vi "correct depth etc 2016.vi"(2 "KPRO Culmulative \ntest report header 2":T1=["Measurement Time", "Current Absolute Depth (Uncorrected)", "Corrected Depth", "Depth Rate", "Flow", "Feet of Stainless Steel Used", "In line Pressure Sensor", "IK", "Corrected Headloss", "Atmospheric Pressure (global)", "Depth to Water Table (global)", "Height of Box (global)", "Resevoir Pressure (global)", "Seconds since Jan 1 1904", "Marker", "Downhole Pressure Sensor (ft/H20)", "Downhole Pressure Sensor (V)", "DHT Depth to Water", "DHT IK", "Current Relative Depth", "Previous Relative Depth"], 3 "New Stainless Feet":i32, 4 "Cumulative_data_in":dbl[][](array[numeric]) format="%.4f", 5 "First Absolute Depth":dbl format="%.2f", 6 "Incorrect Depth":dbl format="%.2f", 7 "Correct Depth":dbl format="%.2f") -> (1 "Cumulative_data_out":dbl[][](array[numeric]) format="%.4f")   [LabVIEW 2016]
uses:
  controls/KPro Header Control 1.ctl
  Kpro Globals.vi
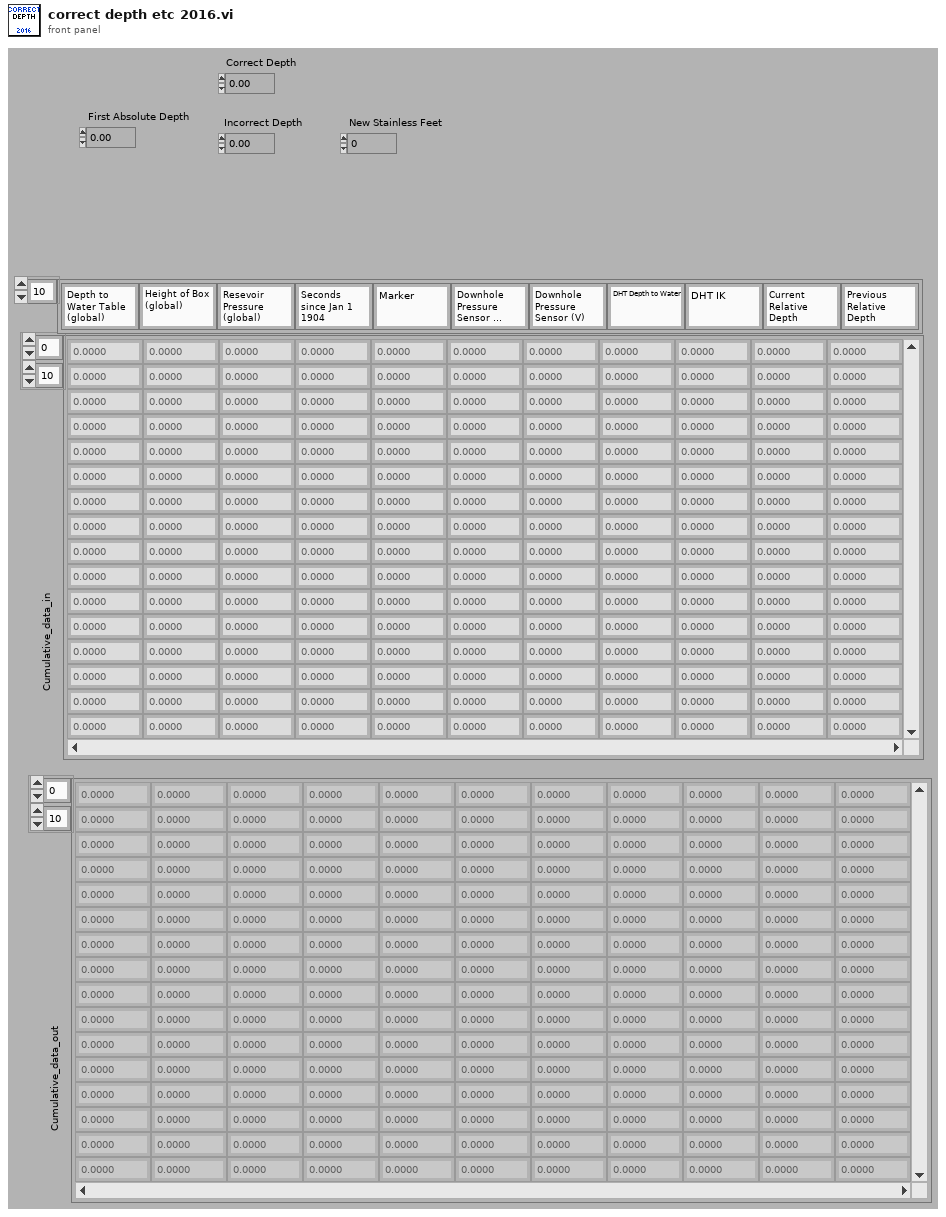
[diagram p1: front panel]
types:
  T1 = typedef "KPro Header Control 1.ctl" = string[]
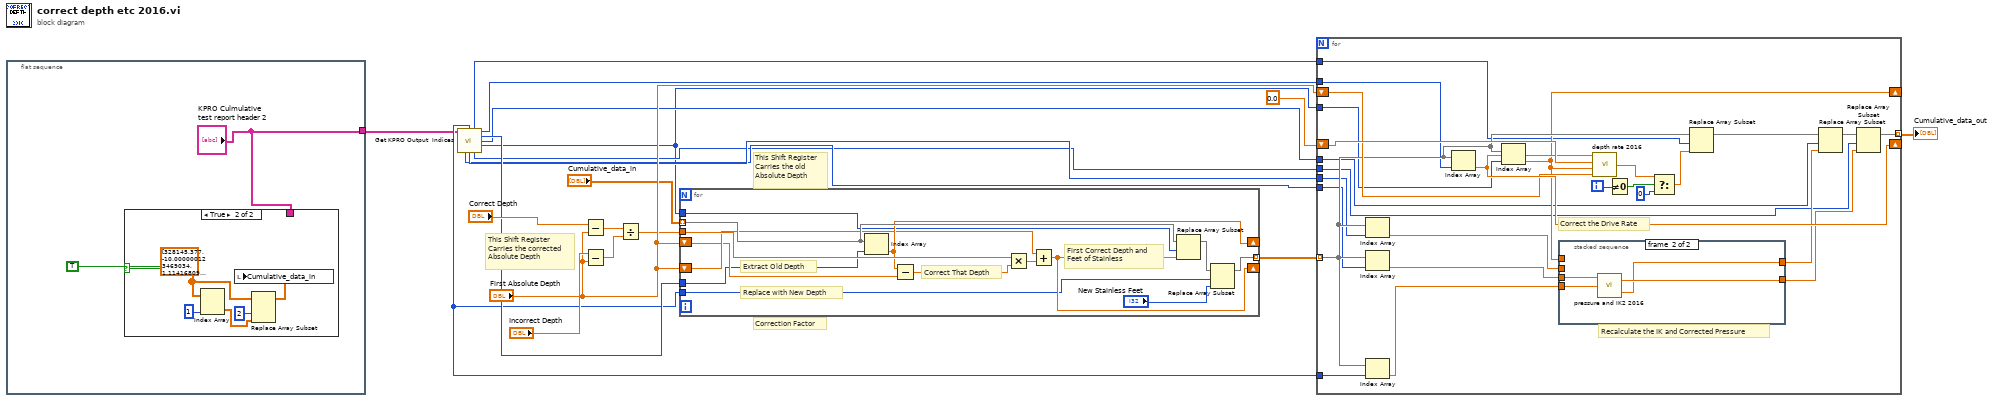
[diagram p0: block diagram]
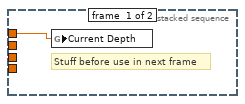
[diagram p3: hidden frame]
diagram:
  # "This Shift Register\nCarries the old\nAbsolute Depth"
  # "This Shift Register\nCarries the corrected \nAbsolute Depth"
  # "Correction Factor"
  n1 = flat-sequence {
    tunnel: ["KPRO Culmulative \ntest report header 2"] -> w1
    frame #0 {
      n2 = case shown="True" TRUE {
        tunnel: "KPRO Culmulative \ntest report header 2" -> [_ _]
        frame False {
        }
        frame True {
          w26 = dbl[][] [[328145.377, -10.000000123469034, 1.1141680910040783, 3.0300636799260526e-09, 0.17185246658325196, 40.0, 0.40080429077148594, 0.003337548440007989, 111.84920433727325, 33.60003003358841, -11.0, 3.0, 65.2670587735176, 3594995318.2992783, 0.0, 1.400799036026001, 0.933866024017334, 0.0, 0.0, 0.030822377713521313, 0.030822501182556142], [328186.551, -9.999996913274128, 1.1141680910040783, 8.864807212475608e-07, 128.47274576377868, 40.0, 53.34394015169144, 2.4950704562609403, 91.90382468603923, 33.60003003358841, -11.0, 3.0, 65.2670587735176, 3594995359.4736333, 0.0, 1.5237629413604736, 1.0158419609069824, 0.0, 0.0, 4.570600807825723, 4.570597721099852], [328188.135, -10.054259825515746, 1.1141680910040783, 0.03425688904074059, 128.03251836585997, 40.0, 53.31440131282807, 2.4865207956457374, 91.99477373239192, 33.60003003358841, -11.0, 3.0, 65.2670587735176, 3594995361.058724, 0.0, 1.7749135494232178, 1.140918254852295, 0.0, 0.0, 4.516337895584106, 4.570600807825723], [328188.59, -10.110125612767536, 1.1141680910040783, 0.12278194999953754, 127.49697208404541, 40.0, 53.265266684055334, 2.4761199460509693, 92.1594728080316, 33.60003003358841, -11.0, 3.0, 65.2670587735176, 3594995361.51275, 0.0, 1.5586717128753662, 1.0304341316223145, 0.0, 0.0, 4.460472108332315, 4.516337895584106], [328189.045, -10.18411276505788, 1.1141680910040783, 0.162609125927821, 127.13181509208678, 40.0, 53.270506743431085, 2.4690282285266294, 92.29050621577258, 33.60003003358841, -11.0, 3.0, 65.2670587735176, 3594995361.966776, 0.0, 1.5038015842437744, 1.0033445358276367, 0.0, 0.0, 4.386484956041971, 4.460472108332315], [328189.502, -10.27626326185862, 1.1141680910040783, 0.20164222494917536, 127.54044259262085, 40.0, 53.24350809955597, 2.476964187224616, 92.28036952761292, 33.60003003358841, -11.0, 3.0, 65.2670587735176, 3594995362.423802, 0.0, 1.500572919845581, 1.001389503479004, 0.0, 0.0, 4.294334459241231, 4.386484956041971], [328189.728, -10.32875241794586, 1.1141680910040783, 0.23225290301599877, 128.94898618888854, 40.0, 53.23854383277893, 2.504319526230641, 92.08152106480425, 33.60003003358841, -11.0, 3.0, 65.2670587735176, 3594995362.6498146, 0.0, 1.5043823719024658, 1.0029568672180176, 0.0, 0.0, 4.241845303153991, 4.294334459241231], [328189.956, -10.38515992558797, 1.1141680910040783, 0.2474013493044673, 129.11139880561828, 40.0, 53.22990716981887, 2.507473743254005, 92.10035452840455, 33.60003003358841, -11.0, 3.0, 65.2670587735176, 3594995362.878828, 0.0, 1.5181667804718018, 1.0096416473388672, 0.0, 0.0, 4.1854377955118816, 4.241845303153991], [328190.182, -10.446334572664895, 1.1141680910040783, 0.2706842791421514, 128.96560032463074, 40.0, 53.249314259529115, 2.5046421895239352, 92.18697543900012, 33.60003003358841, -11.0, 3.0, 65.2670587735176, 3594995363.102841, 0.0, 1.5096580982208252, 1.0051541328430176, 0.0, 0.0, 4.124263148434957, 4.1854377955118816], [328190.408, -10.510489885711667, 1.1141680910040783, 0.2838730665482261, 128.1954029750824, 40.0, 53.24479997015, 2.4896841792399336, 92.40747719898712, 33.60003003358841, -11.0, 3.0, 65.2670587735176, 3594995363.3288536, 0.0, 1.5028095245361328, 1.0011749267578125, 0.0, 0.0, 4.060107835388184, 4.124263148434957], [328190.634, -10.576877951049802, 1.1141680910040783, 0.29375250146469806, 128.28840909576417, 40.0, 53.21862870407105, 2.4914904520224206, 92.45241736162384, 33.60003003358841, -11.0, 3.0, 65.2670587735176, 3594995363.5558667, 0.0, 1.5030255317687988, 1.002260684967041, 0.0, 0.0, 3.993719770050049, 4.060107835388184], [328190.859, -10.643762485376993, 1.1141680910040783, 0.29726459704049235, 128.32822166252134, 40.0, 53.19903291416168, 2.492263652272117, 92.51057835817184, 33.60003003358841, -11.0, 3.0, 65.2670587735176, 3594995363.7818794, 0.0, 1.5053107738494873, 1.0125174522399902, 0.0, 0.0, 3.9268352357228595, 3.993719770050049], [328191.084, -10.710102768198647, 1.1141680910040783, 0.2948457014600877, 128.0759180755615, 40.0, 53.202415002346044, 2.487363661833759, 92.62957959938942, 33.60003003358841, -11.0, 3.0, 65.2670587735176, 3594995364.0058923, 0.0, 1.5080101490020752, 1.003324031829834, 0.0, 0.0, 3.8604949529012047, 3.9268352357228595], [328191.308, -10.776217040952046, 1.1141680910040783, 0.2951530033032548, 128.02690165519715, 40.0, 53.14998537778854, 2.4864117134528345, 92.70603905096685, 33.60003003358841, -11.0, 3.0, 65.2670587735176, 3594995364.2309055, 0.0, 1.8692286014556885, 1.1891350746154785, 0.0, 0.0, 3.7943806801478064, 3.8604949529012047], [328191.532, -10.841864847691852, 1.1141680910040783, 0.29307056581916036, 128.17133135795592, 40.0, 53.12901062488555, 2.4892166841274905, 92.74233173368255, 33.60003003358841, -11.0, 3.0, 65.2670587735176, 3594995364.453918, 0.0, 1.5961782932281494, 1.050705909729004, 0.0, 0.0, 3.728732873407999, 3.7943806801478064], [328191.756, -10.906623677380878, 1.1141680910040783, 0.2891019182708064, 128.19016385841368, 40.0, 53.162047675132754, 2.4895824303036957, 92.80408910768868, 33.60003003358841, -11.0, 3.0, 65.2670587735176, 3594995364.678931, 0.0, 1.5311601161956787, 1.0178089141845703, 0.0, 0.0, 3.6639740437189734, 3.728732873407999], [328191.98, -10.969406508636474, 1.1141680910040783, 0.28028049669249483, 127.66021068763732, 40.0, 53.13022991847991, 2.479290204573289, 92.97819897879899, 33.60003003358841, -11.0, 3.0, 65.2670587735176, 3594995364.902944, 0.0, 1.5098140239715576, 1.0054821968078613, 0.0, 0.0, 3.6011912124633785, 3.6639740437189734], [328192.205, -11.029817314529417, 1.1141680910040783, 0.2684924705936332, 127.99268219947814, 40.0, 53.144266310215, 2.4857471370674986, 92.97240530764333, 33.60003003358841, -11.0, 3.0, 65.2670587735176, 3594995365.127957, 0.0, 2.3484342098236084, 1.429063320159912, 0.0, 0.0, 3.540780406570434, 3.6011912124633785], [328192.43, -11.087652000745138, 1.1141680910040783, 0.25704304987423926, 127.34798765373229, 40.0, 53.148911238193506, 2.473226517967782, 93.1358941073358, 33.60003003358841, -11.0, 3.0, 65.2670587735176, 3594995365.3529696, 0.0, 1.7151710987091064, 1.110060691833496, 0.0, 0.0, 3.482945720354715, 3.540780406570434], [328192.656, -11.14294205188751, 1.1141680910040783, 0.2446462439665919, 127.56047867393492, 40.0, 53.13676184844971, 2.477353308156443, 93.09212873720742, 33.60003003358841, -11.0, 3.0, 65.2670587735176, 3594995365.5789824, 0.0, 1.557053804397583, 1.0291800498962402, 0.0, 0.0, 3.427655669212341, 3.482945720354715], [328192.881, -11.195724693870543, 1.1141680910040783, 0.2345895199488668, 128.11341787910462, 40.0, 53.14984022378921, 2.4880919458863784, 92.9780742114127, 33.60003003358841, -11.0, 3.0, 65.2670587735176, 3594995365.803995, 0.0, 1.5160367488861084, 1.0086207389831543, 0.0, 0.0, 3.374873027229308, 3.427655669212341], [328193.107, -11.246755618921915, 1.1141680910040783, 0.22580055330045729, 128.07636646842957, 40.0, 53.11702090454102, 2.48737237007605, 92.98572443528715, 33.60003003358841, -11.0, 3.0, 65.2670587735176, 3594995366.0310082, 0.0, 1.5068542957305908, 1.0033493041992188, 0.0, 0.0, 3.323842102177937, 3.374873027229308], [328193.561, -11.343619113985696, 1.1141680910040783, 0.2133557160141806, 127.98956704902648, 40.0, 53.12587529850006, 2.485686637700006, 93.00364212464837, 33.60003003358841, -11.0, 3.0, 65.2670587735176, 3594995366.4840345, 0.0, 1.5015649795532227, 0.9996042251586914, 0.0, 0.0, 3.2269786071141557, 3.323842102177937], [328194.013, -11.434393054517109, 1.1141680910040783, 0.2008273020649925, 127.59340015029906, 40.0, 53.0857837638855, 2.47799267647199, 93.08534488670918, 33.60003003358841, -11.0, 3.0, 65.2670587735176, 3594995366.93606, 0.0, 1.5020878314971924, 1.0007939338684082, 0.0, 0.0, 3.136204666582743, 3.2269786071141557], [328194.467, -11.514954006894428, 1.1141680910040783, 0.1774470316575472, 126.88321664619446, 40.0, 53.08781591987609, 2.464200195669304, 93.23149400930774, 33.60003003358841, -11.0, 3.0, 65.2670587735176, 3594995367.389086, 0.0, 1.4985744953155518, 1.5635161399841309, 0.0, 0.0, 3.055643714205424, 3.136204666582743], [328194.924, -11.580785288619992, 1.1141680910040783, 0.1440509446965058, 126.9875269870758, 40.0, 53.088904574871066, 2.4662260078232223, 93.21005319633281, 33.60003003358841, -11.0, 3.0, 65.2670587735176, 3594995367.847112, 0.0, 1.8545379638671875, 1.1820874214172363, 0.0, 0.0, 2.9898124324798587, 3.055643714205424], [328195.377, -11.636100527445473, 1.1141680910040783, 0.12210869498450763, 127.73712186431884, 40.0, 53.05470629262925, 2.480783897290398, 93.05571921234491, 33.60003003358841, -11.0, 3.0, 65.2670587735176, 3594995368.300138, 0.0, 1.5351440906524658, 1.0173463821411133, 0.0, 0.0, 2.9344971936543787, 2.9898124324798587], [328196.061, -11.705785277748106, 1.1141680910040783, 0.10187828991488232, 127.9476069164276, 40.0, 53.03103167533874, 2.4848717295530225, 93.01230164154128, 33.60003003358841, -11.0, 3.0, 65.2670587735176, 3594995368.983177, 0.0, 1.5090909004211426, 1.0038976669311523, 0.0, 0.0, 2.8648124433517452, 2.9344971936543787], [328196.739, -11.758566252899168, 1.1141680910040783, 0.07784804594386162, 127.93236155891418, 40.0, 53.00153638267517, 2.484575649315142, 93.01544755136264, 33.60003003358841, -11.0, 3.0, 65.2670587735176, 3594995369.661216, 0.0, 1.5166218280792236, 1.0088610649108887, 0.0, 0.0, 2.8120314682006833, 2.8648124433517452], [328198.087, -11.815133220799764, 1.1141680910040783, 0.04196362603907464, 128.14737773895263, 40.0, 52.982797001361845, 2.488751480657756, 92.97106135370701, 33.60003003358841, -11.0, 3.0, 65.2670587735176, 3594995371.009293, 0.0, 1.5050232410430908, 1.0118327140808105, 0.0, 0.0, 2.755464500300089, 2.8120314682006833], [328198.99, -11.876306324513752, 1.1141680910040783, 0.06774430090209084, 127.75019605636597, 40.0, 52.945463392734524, 2.4810378113024507, 93.05302338026797, 33.60003003358841, -11.0, 3.0, 65.2670587735176, 3594995371.912345, 0.0, 1.505850076675415, 1.003713607788086, 0.0, 0.0, 2.6942913965861, 2.755464500300089], [328199.444, -11.94183158823649, 1.1141680910040783, 0.144328774711099, 127.59186617469787, 40.0, 52.93785732316971, 2.4779628851167854, 93.08566099936064, 33.60003003358841, -11.0, 3.0, 65.2670587735176, 3594995372.3663707, 0.0, 1.498765468597412, 0.9998078346252441, 0.0, 0.0, 2.628766132863363, 2.6942913965861], [328199.896, -12.03368569761912, 1.1141680910040783, 0.20321705616065797, 126.70874462127685, 40.0, 52.92126622104645, 2.460811772761177, 93.26733698109324, 33.60003003358841, -11.0, 3.0, 65.2670587735176, 3594995372.8183966, 0.0, 1.6621105670928955, 1.0824780464172363, 0.0, 0.0, 2.536912023480733, 2.628766132863363], [328200.124, -12.10274162012736, 1.1141680910040783, 0.3028768531026028, 127.2479724445343, 40.0, 52.89574814796448, 2.4712841216084365, 93.15648107637647, 33.60003003358841, -11.0, 3.0, 65.2670587735176, 3594995373.0464096, 0.0, 1.543135643005371, 1.020904541015625, 0.0, 0.0, 2.4678561009724933, 2.536912023480733], [328200.352, -12.197778576024373, 1.1141680910040783, 0.41682875392915963, 127.6813559513092, 40.0, 52.89947860574722, 2.4797008669465725, 93.06721632514389, 33.60003003358841, -11.0, 3.0, 65.2670587735176, 3594995373.274422, 0.0, 1.51163649559021, 1.0062899589538574, 0.0, 0.0, 2.3728191450754803, 2.4678561009724933], [328200.58, -12.319194814682005, 1.1141680910040783, 0.5325273625269551, 127.44460451698302, 40.0, 52.88404873561859, 2.4751029150171355, 93.1159990491437, 33.60003003358841, -11.0, 3.0, 65.2670587735176, 3594995373.5034356, 0.0, 1.5015113353729248, 1.0010457038879395, 0.0, 0.0, 2.2514029064178467, 2.3728191450754803], [328200.807, -12.472525329462686, 1.1141680910040783, 0.6754648229554004, 127.9867114944458, 40.0, 52.9196550116539, 2.4856311799464716, 93.00423148401865, 33.60003003358841, -11.0, 3.0, 65.2670587735176, 3594995373.728449, 0.0, 1.8673532009124756, 1.1879668235778809, 0.0, 0.0, 2.0980723916371664, 2.2514029064178467], [328201.036, -12.640585082753498, 1.1141680910040783, 0.733885385388227, 127.78493470382689, 40.0, 52.895080439567565, 2.481712470915701, 93.0458597830035, 33.60003003358841, -11.0, 3.0, 65.2670587735176, 3594995373.9594617, 0.0, 1.59521484375, 1.047635555267334, 0.0, 0.0, 1.9300126383463543, 2.0980723916371664], [328201.266, -12.82026018549601, 1.1141680910040783, 0.781196098943757, 127.83215755271911, 40.0, 52.86136116552353, 2.4826295863274637, 93.03612021978995, 33.60003003358841, -11.0, 3.0, 65.2670587735176, 3594995374.1884747, 0.0, 1.525820016860962, 1.0129938125610352, 0.0, 0.0, 1.750337535603841, 1.9300126383463543], [328201.495, -12.998988280741372, 1.1141680910040783, 0.7804720316661126, 127.97738964271545, 40.0, 52.83913808822632, 2.485450140172535, 93.00615538035825, 33.60003003358841, -11.0, 3.0, 65.2670587735176, 3594995374.416488, 0.0, 1.5117781162261963, 1.0070924758911133, 0.0, 0.0, 1.5716094403584797, 1.750337535603841], [328201.724, -13.173716349665323, 1.1141680910040783, 0.7630046678165522, 127.76593700599669, 40.0, 52.830574002265934, 2.4813435164397046, 93.04977749487423, 33.60003003358841, -11.0, 3.0, 65.2670587735176, 3594995374.6455007, 0.0, 1.5158021450042725, 1.0087103843688965, 0.0, 0.0, 1.3968813714345294, 1.5716094403584797], [328201.951, -13.345007225863137, 1.1141680910040783, 0.7545853576547341, 127.06734091758727, 40.0, 52.866223824501034, 2.467776074950949, 93.1936417005304, 33.60003003358841, -11.0, 3.0, 65.2670587735176, 3594995374.873514, 0.0, 1.5053272247314453, 1.0029659271240234, 0.0, 0.0, 1.2255904952367147, 1.3968813714345294], [328202.179, -13.511616958808897, 1.1141680910040783, 0.7307444427356071, 127.14521967887877, 40.0, 52.861927266120915, 2.4692885591382643, 93.17762320562649, 33.60003003358841, -11.0, 3.0, 65.2670587735176, 3594995375.1005273, 0.0, 1.4981188774108887, 0.999793529510498, 0.0, 0.0, 1.0589807622909546, 1.2255904952367147], [328202.405, -13.671555412864684, 1.1141680910040783, 0.7076922745072999, 126.93355464553832, 40.0, 52.84543777179718, 2.465177810448559, 93.22114820598928, 33.60003003358841, -11.0, 3.0, 65.2670587735176, 3594995375.32654, 0.0, 1.5017015933990479, 0.9994425773620605, 0.0, 0.0, 0.8990423082351685, 1.0589807622909546], [328202.631, -13.82470640366872, 1.1141680910040783, 0.6776592514472227, 127.23801340293883, 40.0, 52.83475443744659, 2.4710907069638766, 93.1585305913098, 33.60003003358841, -11.0, 3.0, 65.2670587735176, 3594995375.5535526, 0.0, 1.5003726482391357, 1.000490665435791, 0.0, 0.0, 0.745891317431132, 0.8990423082351685], [328202.857, -13.970626183509825, 1.1141680910040783, 0.6456627425905784, 127.54037179374694, 40.0, 52.80528817558289, 2.476962812238991, 93.09627156564144, 33.60003003358841, -11.0, 3.0, 65.2670587735176, 3594995375.779566, 0.0, 1.5078556537628174, 1.0035624504089355, 0.0, 0.0, 0.599971537590027, 0.745891317431132], [328203.082, -14.109418713315327, 1.1141680910040783, 0.6168556880882833, 127.21967649459839, 40.0, 52.83841231822967, 2.4707345856870457, 93.16230401671167, 33.60003003358841, -11.0, 3.0, 65.2670587735176, 3594995376.0035787, 0.0, 1.503753662109375, 1.0030245780944824, 0.0, 0.0, 0.46117900778452553, 0.599971537590027], [328203.308, -14.242414557139078, 1.1141680910040783, 0.5884771849977928, 127.38029553985595, 40.0, 52.84317336940765, 2.473853969741247, 93.12924219423257, 33.60003003358841, -11.0, 3.0, 65.2670587735176, 3594995376.2295914, 0.0, 1.500307559967041, 1.000640869140625, 0.0, 0.0, 0.32818316396077474, 0.46117900778452553], [328203.534, -14.353985189755756, 1.1141680910040783, 0.49367536563478104, 127.44918284416198, 40.0, 52.81679888772965, 2.475191830754208, 93.11505610825532, 33.60003003358841, -11.0, 3.0, 65.2670587735176, 3594995376.456605, 0.0, 1.498229742050171, 1.2356581687927246, 0.0, 0.0, 0.21661253134409586, 0.32818316396077474], [328203.759, -14.439561824735005, 1.1141680910040783, 0.38034059984873253, 127.76756538009643, 40.0, 52.81354743814468, 2.481375141109076, 93.0494417023131, 33.60003003358841, -11.0, 3.0, 65.2670587735176, 3594995376.6826177, 0.0, 1.6151704788208008, 1.0583596229553223, 0.0, 0.0, 0.1310358963648478, 0.21661253134409586], [328203.984, -14.498762263679502, 1.1141680910040783, 0.2631130620027768, 127.96181389045715, 40.0, 52.80010617780685, 2.4851476433350723, 93.00936983684407, 33.60003003358841, -11.0, 3.0, 65.2670587735176, 3594995376.9076304, 0.0, 1.890188455581665, 1.1963868141174316, 0.0, 0.0, 0.07183545742034911, 0.1310358963648478]] ("Cumulative_data_from_file")
          n3 = Index Array(array=w26, index (col)=1 ("disabled index (col)")) -> (element=w23:dbl[])  [unwired: 1 in]
          n4 = Replace Array Subset(array=w26, new element=w23, index (col)=2 ("disabled index (col)")) -> (w25:dbl[][])  [unwired: 1 in]
          n5 = local write "Cumulative_data_in"(w25) -> ()
        }
      }
    }
  }
  n6 = call "Get KPRO Output  Indices.vi"("KPRO Culmulative \ntest report header 2"=w1) -> ("Feet of Stainless Steel"=w8:i32, "Depth Rate Index"=w2:i32, "Measurement Time Index"=w9:i32, "Uncorrected Depth Index"=w10:i32, "Headloss index"=w4:i32, "Corrected Depth Index"=w3:i32, "Flow Index"=w6:i32, "Pressure Index"=w7:i32, "IK index"=w5:i32)  [unwired: 3 in, 3 out]
  n7 = Subtract(x="Correct Depth", y="First Absolute Depth") -> (x-y=w17:dbl)
  n8 = Subtract(x="Incorrect Depth", y="First Absolute Depth") -> (x-y=w15:dbl)
  n9 = Divide(x=w17, y=w15) -> (x/y=w13:dbl)
  n10 = for {
    tunnel: "Cumulative_data_in" -> [w41] mode=indexing
    shift-right: [w37] -> _
    shift-left: "First Absolute Depth" -> [w35]
    tunnel: [w33] -> w19 mode=indexing
    tunnel: w13 -> [w39]
    shift-right: [w36] -> _
    shift-left: "First Absolute Depth" -> [w34]
    tunnel: w10 -> [w30]
    tunnel: w3 -> [w29]
    tunnel: w8 -> [w28]
    # "Replace with New Depth"
    # "Correct That Depth"
    # "Extract Old Depth"
    # "First Correct Depth and \nFeet of Stainless"
    n11 = Index Array(array=w41, index=w30) -> (element=w36:dbl)
    n12 = Subtract(x=w36, y=w34) -> (x-y=w40:dbl)
    n13 = Multiply(x=w39, y=w40) -> (x*y=w38:dbl)
    n14 = Add(x=w35, y=w38) -> (x+y=w37:dbl)
    n15 = Replace Array Subset(array=w41, new element=w37, index=w29) -> (w32:dbl[])
    n16 = Replace Array Subset(array=w32, new element="New Stainless Feet", index=w28) -> (w33:dbl[])
  }
  n17 = for {
    tunnel: w19 -> [w54] mode=indexing
    shift-right: [w50] -> _
    shift-left: "First Absolute Depth" -> [w60]
    shift-right: [w61] -> _
    shift-left: 0.0 -> [w62]
    tunnel: [w57] -> w11 mode=indexing
    tunnel: w9 -> [w43]
    tunnel: w8 -> [w49]
    tunnel: w7 -> [w48]
    tunnel: w6 -> [w47]
    tunnel: w5 -> [w46]
    tunnel: w4 -> [w45]
    tunnel: w3 -> [w44]
    tunnel: w2 -> [w42]
    i -> [w67]
    # "Recalculate the IK and Corrected Pressure"
    # "Correct the Drive Rate"
    n18 = Index Array(array=w54, index=w48) -> (element=w51:dbl)
    n19 = Index Array(array=w54, index=w47) -> (element=w53:dbl)
    n20 = Index Array(array=w54, index=w49) -> (element=w52:dbl)
    n21 = Index Array(array=w54, index=w43) -> (element=w61:dbl)
    n22 = Index Array(array=w54, index=w44) -> (element=w50:dbl)
    n23 = stacked-sequence {
      tunnel: [_ w70] -> w56
      tunnel: [_ w69] -> w55
      tunnel: w53 -> [_ w72]
      tunnel: w52 -> [_ w71]
      tunnel: w51 -> [_ _]
      tunnel: w50 -> [w68 _]
      frame #0 {
        # "Stuff before use in next frame"
        n24 = global write "Kpro Globals.vi" "Current Depth"(w68) -> ()
      }
      frame #1 {
        n25 = call "pressure and IK2 2016.vi"("Ft. of SS"=w71, "flow"=w72) -> ("Corrected Headloss"=w69:dbl, "IK"=w70:dbl)  [unwired: 1 in]
      }
    }
    n26 = call "depth rate 2016.vi"("Depth Last"=w60, "Depth Current"=w50, "Time Last"=w62, "Time Current"=w61) -> ("Depth Rate"=w64:dbl)
    n27 = Not Equal To 0?(x=w67) -> (x != 0?=w66:bool)
    n28 = Select(t=w64, s=w66, f=0) -> (s? t:f=w63:dbl)
    n29 = Replace Array Subset(array=w54, new element=w63, index=w42) -> (w59:dbl[])
    n30 = Replace Array Subset(array=w59, new element=w55, index=w45) -> (w58:dbl[])
    n31 = Replace Array Subset(array=w58, new element=w56, index=w46) -> (w57:dbl[])
  }
  "Cumulative_data_out" <- w11
